vi "NicmosMaskGlobal.vi"() -> ()   [LabVIEW 2009]
panel:
  out "Mask List":bool[][][](array[boolean])
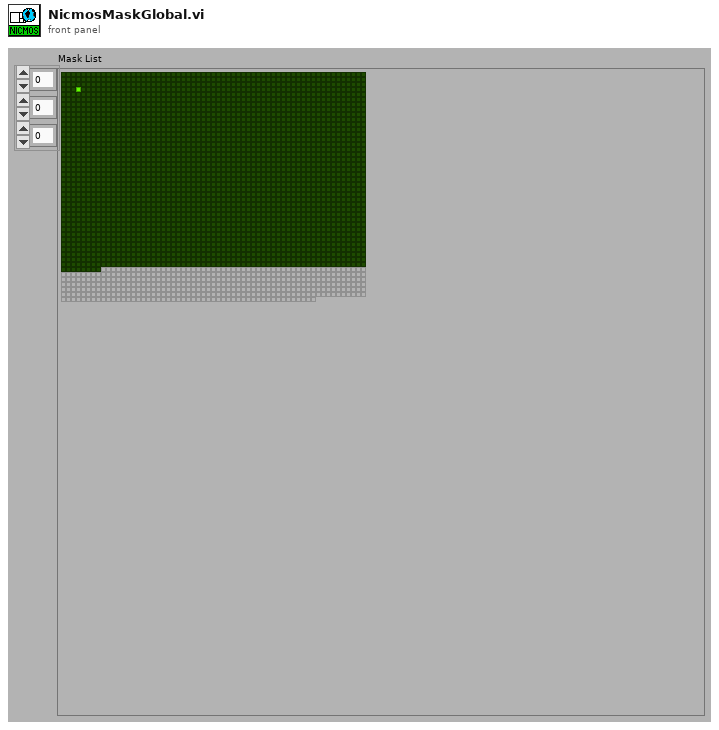
[diagram p1: front panel]
diagram:
